vi "svx_Orbit Update Pair.vi"(6 "State in":T1={"X Scale"={"Name"="Horizontal", "FString"="%#.2g", "Major Color"=16777238, "Minor Color"=16777216, "Scale Visible"=TRUE, " Label Visible"=TRUE, "Grid Style"=1}, "Y Scale"={"Name"="Vertical", "FString"="%#.2g", "Major Color"=16777238, "Minor Color"=16777216, "Scale Visible"=TRUE, " Label Visible"=TRUE, "Grid Style"=1}, "Plot"={"Point Style"=0, "Line Width"=0, "Line Style"=0, "Plot Color"=9727, "Point/fill"=0}, "Arrow/Crosshair Color"=9727, "Tacho Point Color"=16711680, "Container Bounds"={"Width"=563, "Height"=294}, "Axis Maximum"=10.0, "Probe Angles"={"Angle X"=0.0, "Angle Y"=1.5707963267948966}, "Background Color"=16777226, "Cursor"={"Cursor Point Style"=13, "Cursor Style"=4, "Cursor Line Width"=1, "Cursor Line Style"=0, "Cursor Color"=9727, "Cursor Name Visible"=TRUE, "Cursor Visible"=TRUE, "Cursor Position"={"X"=0.0, "Y"=0.0}, "Cursor Index"=0, "Cursor Lock"=FALSE}, "Elliptical Info"=[], "Legend Visible"=TRUE, "Scale Range Change"=refnum, "Strings[]"={"Custom pair name"=FALSE, "Row Strings []"=[], "Column Strings []"=[]}, "Index"=[{"pair index"=0, "order index"=0}], " Parents Tags"=[], "Children Tags"=[], "Open?"=[], "Label"="", "Legend Width"=120, "Pair Strings Changed?"=FALSE, "Size"=[], "Legend Background"=16777226, "Legend Font"=16777222, "Cursor Release"=refnum, "Autoscale"=TRUE, "Precession Direction"=[], "Item Width"=0, "User Pair Strings []"=[], "Users Order Strings []"=[], "Autoscale Once"=TRUE, "Property Write"=refnum} caption="State" {"Index"."order index" min=0; "Index"."pair index" min=0; "Axis Maximum" min=0.0}, 10 "Label.Text":string, 11 "orbit plot":T3) -> (0 "update tree?":bool, 4 "State out":T1={"X Scale"={"Name"="Horizontal", "FString"="%#.2g", "Major Color"=16777238, "Minor Color"=16777216, "Scale Visible"=TRUE, " Label Visible"=TRUE, "Grid Style"=1}, "Y Scale"={"Name"="Vertical", "FString"="%#.2g", "Major Color"=16777238, "Minor Color"=16777216, "Scale Visible"=TRUE, " Label Visible"=TRUE, "Grid Style"=1}, "Plot"={"Point Style"=0, "Line Width"=0, "Line Style"=0, "Plot Color"=9727, "Point/fill"=0}, "Arrow/Crosshair Color"=9727, "Tacho Point Color"=16711680, "Container Bounds"={"Width"=563, "Height"=294}, "Axis Maximum"=10.0, "Probe Angles"={"Angle X"=0.0, "Angle Y"=1.5707963267948966}, "Background Color"=16777226, "Cursor"={"Cursor Point Style"=13, "Cursor Style"=4, "Cursor Line Width"=1, "Cursor Line Style"=0, "Cursor Color"=9727, "Cursor Name Visible"=TRUE, "Cursor Visible"=TRUE, "Cursor Position"={"X"=0.0, "Y"=0.0}, "Cursor Index"=0, "Cursor Lock"=FALSE}, "Elliptical Info"=[], "Legend Visible"=TRUE, "Scale Range Change"=refnum, "Strings[]"={"Custom pair name"=FALSE, "Row Strings []"=[], "Column Strings []"=[]}, "Index"=[{"pair index"=0, "order index"=0}], " Parents Tags"=[], "Children Tags"=[], "Open?"=[], "Label"="", "Legend Width"=120, "Pair Strings Changed?"=FALSE, "Size"=[], "Legend Background"=16777226, "Legend Font"=16777222, "Cursor Release"=refnum, "Autoscale"=TRUE, "Precession Direction"=[], "Item Width"=0, "User Pair Strings []"=[], "Users Order Strings []"=[], "Autoscale Once"=TRUE, "Property Write"=refnum} caption="State" {"Index"."order index" min=0; "Index"."pair index" min=0; "Axis Maximum" min=0.0})   [LabVIEW 2017, in "SVX Orbit.xctl"]
uses:
  <vilib>/addons/_XControls/Orbit Plot/SVX Orbit.xctl
  <vilib>/addons/_XControls/Orbit Plot/subVIs/svx_Orbit Data.ctl
  <vilib>/addons/_XControls/Orbit Plot/subVIs/svx_Orbit Internal State.ctl
  <vilib>/addons/_XControls/Orbit Plot/subVIs/svx_Orbit Bounds.ctl
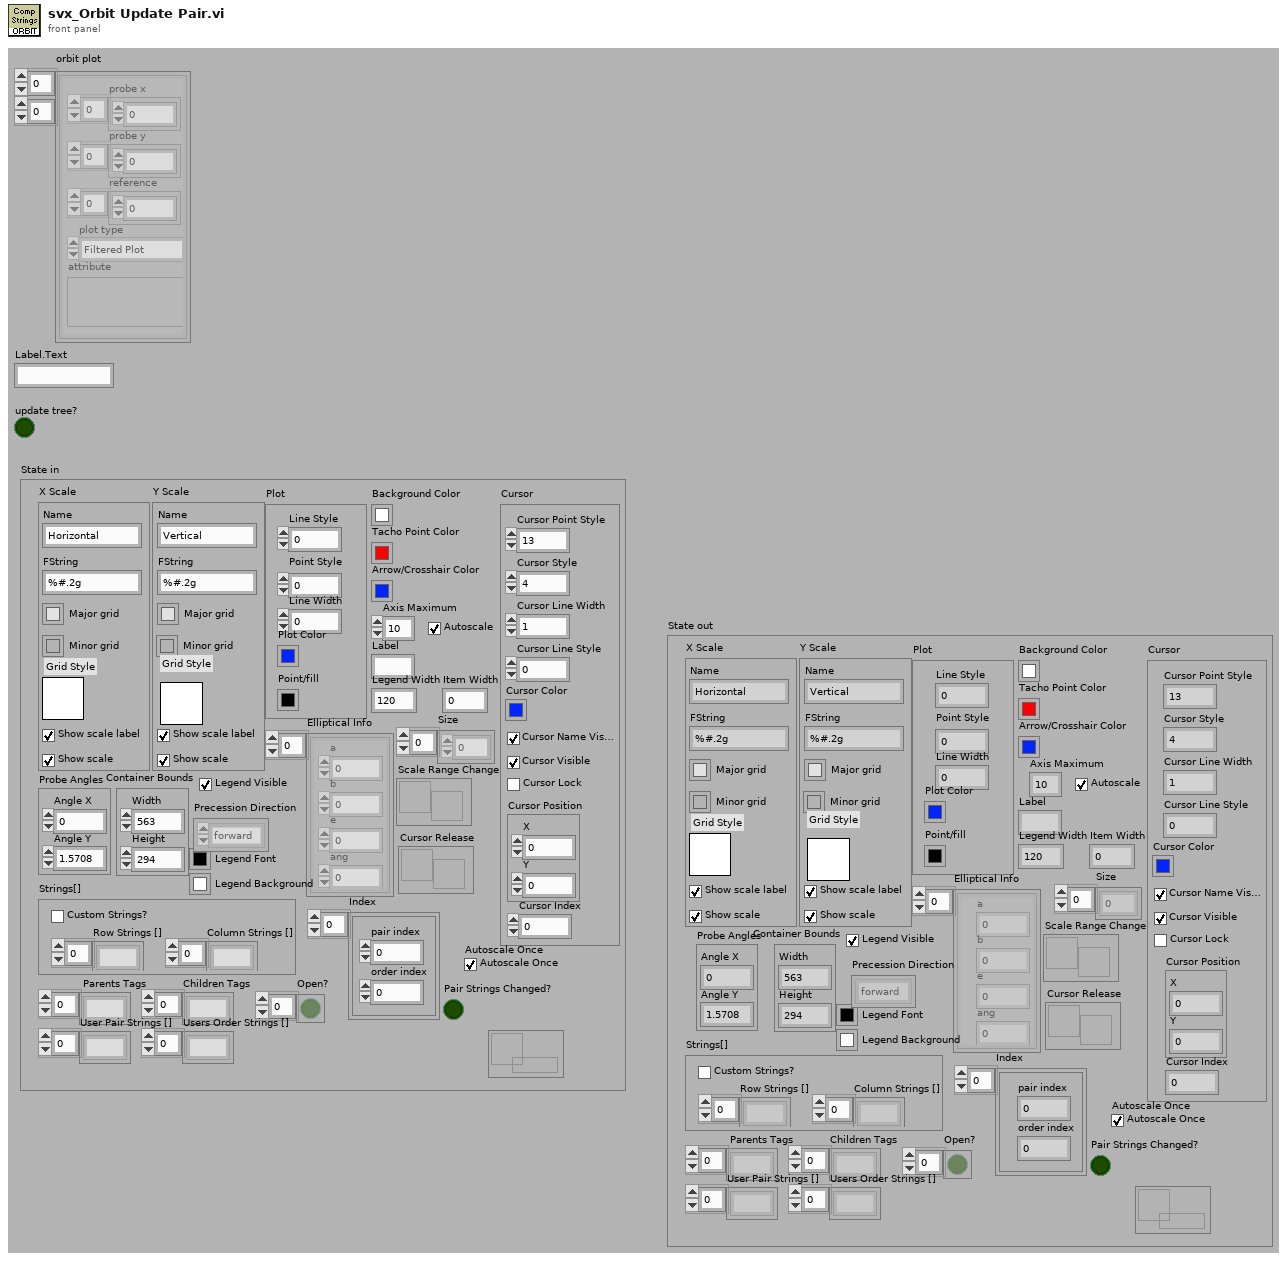
[diagram p1: front panel]
types:
  T1 = typedef "SVX Orbit.xctl/svx_Orbit Internal State.ctl" = cluster{"X Scale":cluster{"Name":string, "FString":string, "Major Color":u32, "Minor Color":u32, "Scale Visible":bool, " Label Visible":bool, "Grid Style":u16}, "Y Scale":cluster{"Name":string, "FString":string, "Major Color":u32, "Minor Color":u32, "Scale Visible":bool, " Label Visible":bool, "Grid Style":u16}, "Plot":cluster{"Point Style":u8, "Line Width":u8, "Line Style":u8, "Plot Color":u32, "Point/fill":u32}, "Arrow/Crosshair Color":u32, "Tacho Point Color":u32, "Container Bounds":T2, "Axis Maximum":dbl, "Probe Angles":cluster{"Angle X":dbl, "Angle Y":dbl}, "Background Color":u32, "Cursor":cluster{"Cursor Point Style":u8, "Cursor Style":u8, "Cursor Line Width":u8, "Cursor Line Style":u8, "Cursor Color":u32, "Cursor Name Visible":bool, "Cursor Visible":bool, "Cursor Position":cluster{"X":dbl, "Y":dbl}, "Cursor Index":i32, "Cursor Lock":bool}, "Elliptical Info":cluster{"a":dbl, "b":dbl, "e":dbl, "ang":dbl}[], "Legend Visible":bool, "Scale Range Change":refnum<user-event>, "Strings[]":cluster{"Custom pair name":bool, "Row Strings []":string[], "Column Strings []":string[]}, "Index":cluster{"pair index":i32, "order index":i32}[], " Parents Tags":string[], "Children Tags":string[], "Open?":bool[], "Label":string, "Legend Width":u32, "Pair Strings Changed?":bool, "Size":i32[], "Legend Background":u32, "Legend Font":u32, "Cursor Release":refnum<user-event>, "Autoscale":bool, "Precession Direction":enum16{"forward", "backward"}[], "Item Width":u32, "User Pair Strings []":string[], "Users Order Strings []":string[], "Autoscale Once":bool, "Property Write":refnum<queue>}
  T2 = typedef "SVX Orbit.xctl/svx_Orbit Bounds.ctl" = cluster{"Width":u32, "Height":u32}
  T3 = typedef "SVX Orbit.xctl/svx_Orbit Data.ctl" = cluster{"probe x":dbl[], "probe y":dbl[], "reference":dbl[], "plot type":enum16{"Filtered Plot", "Unfiltered Plot"}, "attribute":variant}[][]
  T4 = cluster{"probe x":dbl[], "probe y":dbl[], "reference":dbl[], "plot type":enum16{"Filtered Plot", "Unfiltered Plot"}, "attribute":variant}
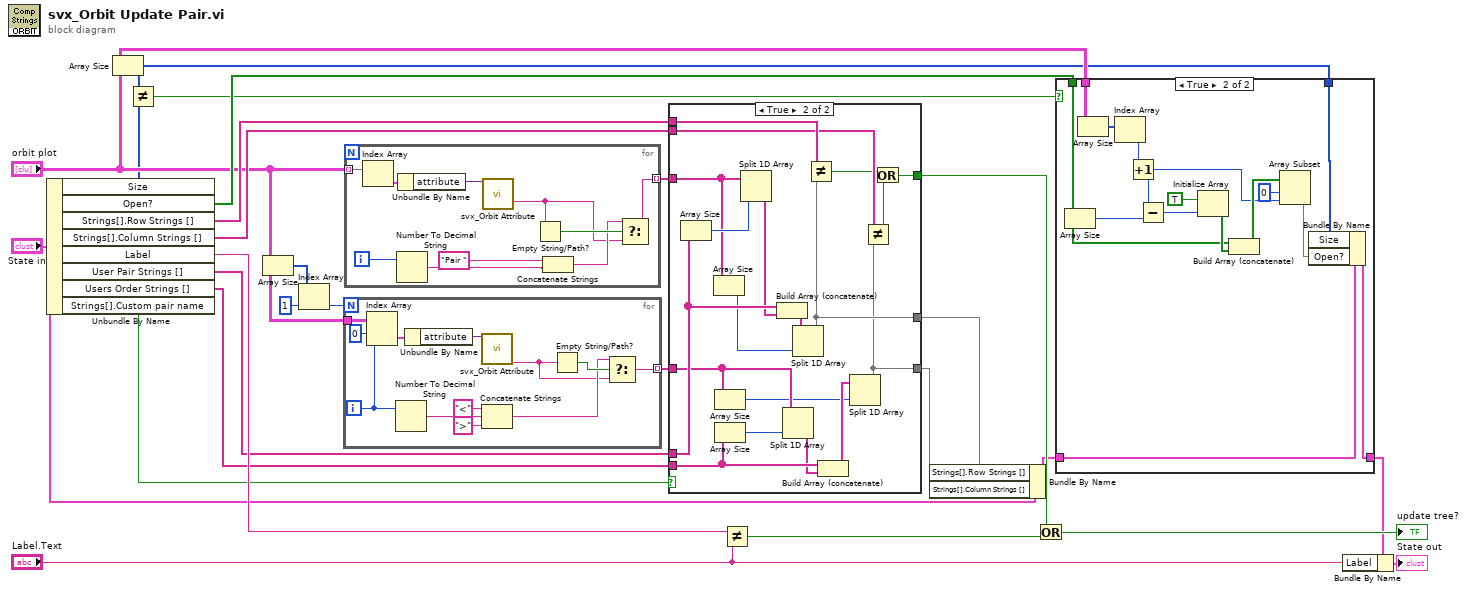
[diagram p0: block diagram]
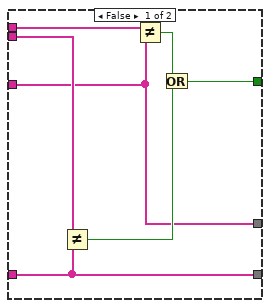
[diagram p2: hidden frame]
diagram:
  n1 = Unbundle By Name("State in") -> ("Size"=w19:i32[], "Open?"=w21:bool[], "Strings[].Row Strings []"=w26:string[], "Strings[].Column Strings []"=w25:string[], "Label"=w10:string, "User Pair Strings []"=w6:string[], "Users Order Strings []"=w5:string[], "Strings[].Custom pair name"=w7:bool)
  n2 = Array Size(array="orbit plot") -> (size(s)=w17:i32[])
  n3 = Not Equal?(x=w17, y=w19) -> (x != y?=w18:bool)
  n4 = Array Size(array="orbit plot") -> (size(s)=w13:i32[])
  n5 = Index Array(array=w13, index=1) -> (element=w11:i32)
  n6 = for {
    N: w11 -> [_]
    tunnel: "orbit plot" -> [w38]
    tunnel: [w31] -> w8 mode=indexing
    i -> [w37]
    n7 = Index Array(array=w38, index (row)=0 ("disabled index (row)"), index (col)=w37) -> (element=w35:T4)
    n8 = Number To Decimal String(number=w37) -> (decimal integer string=w32:string)  [unwired: 1 in]
    n9 = Unbundle By Name(w35) -> ("attribute"=w30:variant)
    n10 = call <vilib>:"svx_Orbit Attribute.vi"("attribute"=w30) -> ("order"=w27:string)  [unwired: 13 in, 5 out]
    n11 = Concatenate Strings("<" ("string"), w32, ">" ("string")) -> (w28:string)
    n12 = Empty String/Path?(string/path=w27) -> (empty?=w29:bool)
    n13 = Select(t=w28, s=w29, f=w27) -> (s? t:f=w31:string)
  }
  n14 = for {
    tunnel: "orbit plot" -> [w47] mode=indexing
    tunnel: [w43] -> w9 mode=indexing
    i -> [w45]
    n15 = Index Array(array=w47) -> (element=w46:T4)  [unwired: 1 in]
    n16 = Number To Decimal String(number=w45) -> (decimal integer string=w44:string)  [unwired: 1 in]
    n17 = Unbundle By Name(w46) -> ("attribute"=w42:variant)
    n18 = call <vilib>:"svx_Orbit Attribute.vi"("attribute"=w42) -> ("pair"=w39:string)  [unwired: 13 in, 5 out]
    n19 = Empty String/Path?(string/path=w39) -> (empty?=w41:bool)
    n20 = Concatenate Strings("Pair " ("string"), w44) -> (w40:string)
    n21 = Select(t=w40, s=w41, f=w39) -> (s? t:f=w43:string)
  }
  n22 = case shown="True" w7 {
    tunnel: w26 -> [w55 w71]
    tunnel: w25 -> [w54 w67]
    tunnel: [w53 w64] -> w23
    tunnel: w9 -> [w49 w58]
    tunnel: w8 -> [w50 w60]
    tunnel: w6 -> [_ w74]
    tunnel: w5 -> [_ w70]
    tunnel: [w49 w63] -> w2
    tunnel: [w50 w62] -> w1
    frame False {
      n23 = Not Equal?(x=w54, y=w50) -> (x != y?=w51:bool)
      n24 = Not Equal?(x=w55, y=w49) -> (x != y?=w52:bool)
      n25 = Or(x=w52, y=w51) -> (x .or. y?=w53:bool)
    }
    frame True {
      n26 = Array Size(array=w74) -> (size(s)=w61:i32)
      n27 = Array Size(array=w58) -> (size(s)=w56:i32)
      n28 = Array Size(array=w60) -> (size(s)=w57:i32)
      n29 = Array Size(array=w70) -> (size(s)=w59:i32)
      n30 = Split 1D Array(array=w58, index=w61) -> (second subarray=w73:string[])  [unwired: 1 out]
      n31 = Build Array (concatenate)(w74, w73) -> (w72:string[])
      n32 = Split 1D Array(array=w60, index=w59) -> (second subarray=w69:string[])  [unwired: 1 out]
      n33 = Split 1D Array(array=w72, index=w56) -> (first subarray=w63:string[])  [unwired: 1 out]
      n34 = Not Equal?(x=w71, y=w63) -> (x != y?=w66:bool)
      n35 = Build Array (concatenate)(w70, w69) -> (w68:string[])
      n36 = Split 1D Array(array=w68, index=w57) -> (first subarray=w62:string[])  [unwired: 1 out]
      n37 = Not Equal?(x=w67, y=w62) -> (x != y?=w65:bool)
      n38 = Or(x=w66, y=w65) -> (x .or. y?=w64:bool)
    }
  }
  n39 = Not Equal?(x=w10, y="Label.Text") -> (x != y?=w24:bool)
  n40 = Bundle By Name(cluster="State in", "Strings[].Row Strings []"=w2, "Strings[].Column Strings []"=w1) -> (w3:T1)
  n41 = Or(x=w23, y=w24) -> (x .or. y?=→"update tree?":bool)
  n42 = case shown="True" w18 {
    tunnel: w3 -> [w75 w90]
    tunnel: [w75 w89] -> w16
    tunnel: w21 -> [_ w82]
    tunnel: "orbit plot" -> [_ w77]
    tunnel: w17 -> [_ w76]
    frame False {
    }
    frame True {
      n43 = Array Size(array=w82) -> (size(s)=w88:i32)
      n44 = Array Size(array=w77) -> (size(s)=w81:i32[])
      n45 = Index Array(array=w81) -> (element=w79:i32)  [unwired: 1 in]
      n46 = Increment(x=w79) -> (x+1=w78:i32)
      n47 = Subtract(x=w78, y=w88) -> (x-y=w87:i32)
      n48 = Initialize Array(TRUE ("x .or. y?"), w87) -> (w85:bool[])
      n49 = Build Array (concatenate)(w82, w85) -> (w84:bool[])
      n50 = Array Subset(array=w84, index=0, length=w78) -> (w80:bool[])
      n51 = Bundle By Name(cluster=w90, "Size"=w76, "Open?"=w80) -> (w89:T1)
    }
  }
  n52 = Bundle By Name(cluster=w16, "Label"="Label.Text") -> (→"State out":T1)
